vi "EpochNotTimestamp.vi"(1 "Epoch (UTC)":T1=enum."UTC", 2 "Epoch Time":ext format="%#.6f") -> (7 "Not a Timestamp?":bool)   [LabVIEW 2018]
doc: "LabVIEW Timestamp is from 1600-01-01 to 3000-12-31.\nAny values outside this range cannot map to a timestamp and will display as \"00:00:00.000 PM YYYY-MM-DD\""
uses:
  Epochs -- enum.ctl
  epoch/Epoch.lvclass
  epoch.UTC/Epoch.UTC.lvclass
  C:/Users/Fujitsu/Documents/avril/Epoch Date & Time/epoch/Epoch.lvclass
  epoch.UNIX/Epoch.UNIX.lvclass
  epoch.GPS/Epoch.GPS.lvclass
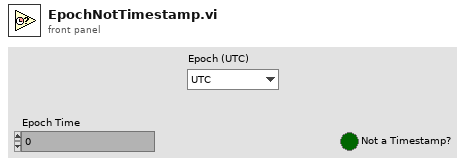
[diagram p1: front panel]
types:
  T1 = typedef "Epochs -- enum.ctl" = enum16{"Local", "UTC", "Unix", "GPS"}
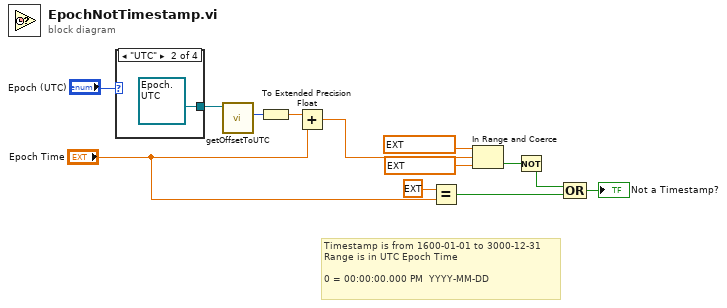
[diagram p0: block diagram]
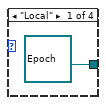
[diagram p2: hidden frame]
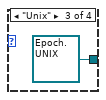
[diagram p3: hidden frame]
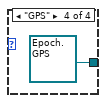
[diagram p4: hidden frame]
diagram:
  # "Timestamp is from 1600-01-01 to 3000-12-31\nRange is in UTC Epoch Time\n\n0 = 00:00:00.000 PM  YYYY-MM-DD"
  n1 = case shown="\"UTC\"" "Epoch (UTC)" {
    tunnel: [refnum<class "Epoch.lvclass"> refnum ("Epoch.lvclass") refnum<class "Epoch.UTC.lvclass"> refnum ("Epoch.UTC.lvclass") refnum<class "Epoch.UNIX.lvclass"> refnum ("Epoch.UNIX.lvclass") refnum<class "Epoch.GPS.lvclass"> refnum ("Epoch.GPS.lvclass")] -> w7
    frame "Local" {
    }
    frame "UTC" {
    }
    frame "Unix" {
    }
    frame "GPS" {
    }
  }
  n2 = call-dynamic "getOffsetToUTC.vi"("Epoch"=w7) -> ("Offset to UTC"=w10:i64)  [unwired: 10 in]
  n3 = To Extended Precision Float(1:w10) -> (0:w9:ext)
  n4 = Add(x=w9, y="Epoch Time") -> (x+y=w4:ext)
  n5 = Equal?(x=ext 0.0 ("y"), y="Epoch Time") -> (x = y?=w1:bool)
  n6 = In Range and Coerce(upper limit=ext 34618060800.0 ("y"), x=w4, lower limit=ext -9593251200.0 ("y")) -> (In Range?=w13:bool)  [unwired: 1 out]
  n7 = Not(x=w13) -> (.not. x?=w6:bool)
  n8 = Compound Arithmetic op=OR(w6, w1) -> (→"Not a Timestamp?":bool)
